vi "HP-connect.vi"(8 "error in (no error)":errorcluster, 11 "HP-S-Serial in":refnum<class "HP-S-Serial.lvclass">) -> (0 "error out":errorcluster, 3 "HP-S-Serial out":refnum<class "HP-S-Serial.lvclass">)   [LabVIEW 2020, in "HP-S-Serial.lvclass"]
uses:
  HP-S-Serial.lvclass
  HP-S-Serial.lvclass/HP-S-Serial.ctl
  <vilib>/Instr/_visa.llb/VISA Configure Serial Port (Instr).vi
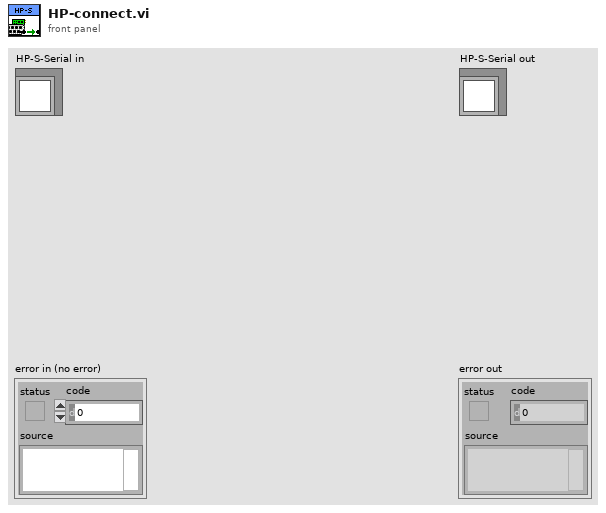
[diagram p1: front panel]
types:
  T1 = typedef "HP-S-Serial.lvclass/HP-S-baudrate.ctl" = u32
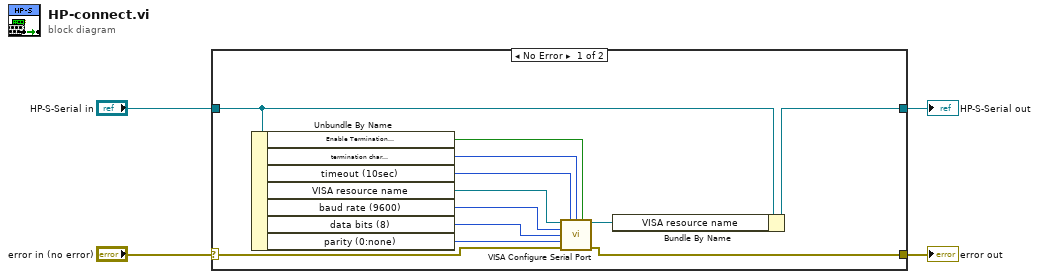
[diagram p0: block diagram]
diagram:
  n1 = case shown="No Error" "error in (no error)" {
    selector: "error in (no error)" -> [w6 w18]
    tunnel: [w5 w18] -> w3
    tunnel: [w8 w17] -> w1
    tunnel: "HP-S-Serial in" -> [w16 w17]
    frame No Error {
      n2 = Unbundle By Name(w16) -> ("Enable Termination\nChar (T)"=w14:bool, "termination char\n(0xA = '\\n' = LF)"=w13:u8, "timeout (10sec)"=w12:u32, "VISA resource name"=w15:refnum<visa-resource-name>, "baud rate (9600)"=w9:T1, "data bits (8)"=w10:u16, "parity (0:none)"=w11:enum16{"None", "Odd", "Even", "Mark", "Space"})
      n3 = call-poly "VISA Configure Serial Port"("VISA resource name"=w15, "timeout (10sec)"=w12, "termination char\n(0xA = '\\n' = LF)"=w13, "Enable Termination\nChar (T)"=w14, "baud rate (9600)"=w9, "data bits (8)"=w10, "parity (0:none)"=w11, "error in (no error)"=w6) -> ("VISA resource name out"=w7:refnum<visa-resource-name>, "error out"=w5:errorcluster)  [unwired: 2 in, 4 out]
      n4 = Bundle By Name(cluster=w16, "VISA resource name"=w7) -> (w8:refnum<class "HP-S-Serial.lvclass">)
    }
    frame Error {
    }
  }
  "error out" <- w3
  "HP-S-Serial out" <- w1
